vi "Position_Two_Scoring.vi"(11 "Stop":string) -> (3 "String":string)   [LabVIEW 2012, in "Serenity_mk2.lvrbt"]
uses:
  Serenity_mk2.lvrbt
  auto_drive_TYP.ctl
  State_Typ.ctl
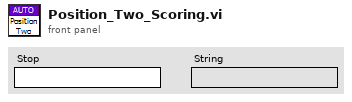
[diagram p1: front panel]
types:
  T1 = typedef "auto_drive_TYP.ctl" = cluster{"Left X":i8, "Left Y":i8, "Right Y":i8, "Power (100)":i8, "Wait (ms)":u32, "Enc/Deg Target":i32, "Move Type":enum16{"Relative Degrees", "Wait", "Encoder"}}
  T2 = typedef "State_Typ.ctl" = enum16{"Stop", "Check for Position 3", "Check for Position 2", "Move", "Reset Enc", "Read Enc", "Lift", "Dump Close"}
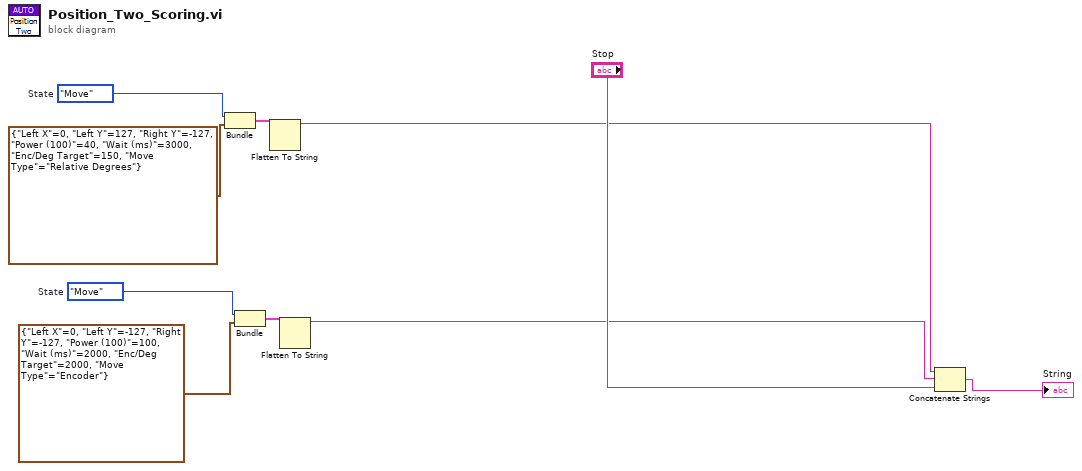
[diagram p0: block diagram]
diagram:
  w7 = State_Typ."Move"  # State
  w3 = State_Typ."Move"  # State
  n1 = Bundle("State"=w3, "Drive Control"=T1 {"Left X"=0, "Left Y"=127, "Right Y"=-127, "Power (100)"=40, "Wait (ms)"=3000, "Enc/Deg Target"=150, "Move Type"=enum."Relative Degrees"}) -> (w2:cluster{"State":T2, "Drive Control":T1})  [unwired: 1 in]
  n2 = Bundle("State"=w7, "Drive Control"=T1 {"Left X"=0, "Left Y"=-127, "Right Y"=-127, "Power (100)"=100, "Wait (ms)"=2000, "Enc/Deg Target"=2000, "Move Type"=enum."Encoder"}) -> (w6:cluster{"State":T2, "Drive Control":T1})  [unwired: 1 in]
  n3 = Flatten To String(anything=w2) -> (data string=w4:string)  [unwired: 3 in, 2 out]
  n4 = Flatten To String(anything=w6) -> (data string=w8:string)  [unwired: 3 in, 2 out]
  n5 = Concatenate Strings(w4, w8, "Stop") -> (→"String":string)
